vi "__init__.vi"(8 "error in (no error)":errorcluster, 11 "Frequencies":dbl[](array[numeric])) -> (0 "error out":errorcluster, 3 "Resonance Curve Data out":refnum<class "Resonance Curve Data.lvclass">)   [LabVIEW 2020, in "Resonance Curve Data.lvclass"]
uses:
  Resonance Curve Data.lvclass
  Resonance Curve Data.lvclass/Resonance Curve Data.ctl
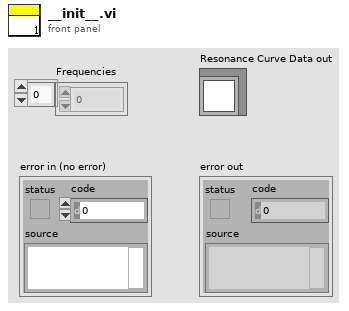
[diagram p1: front panel]
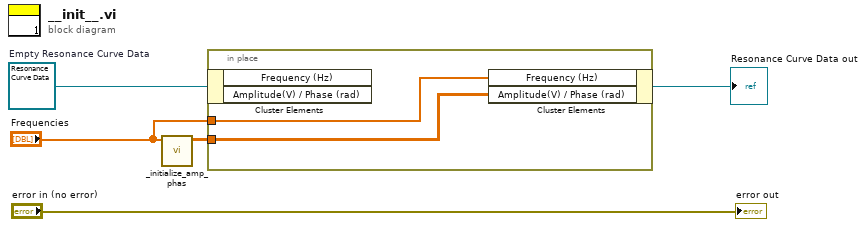
[diagram p0: block diagram]
diagram:
  w5 = refnum<class "Resonance Curve Data.lvclass"> refnum  # Empty Resonance Curve Data
  n1 = call "_initialize_amp_phas.vi"("Measurement Frequencies"="Frequencies") -> ("Initialized Amp/Phas"=w4:dbl[][])  [unwired: 10 in]
  n2 = in-place {
    in-place-border: w4 -> [w7]
    in-place-border: "Frequencies" -> [w6]
    n3 = in-place-cluster #1(w5) -> ()  [unwired: 2 out]
    n4 = in-place-cluster #1("Frequency (Hz)"=w6, "Amplitude(V) / Phase (rad)"=w7) -> (→"Resonance Curve Data out":refnum<class "Resonance Curve Data.lvclass">)
  }
  "error out" <- "error in (no error)"
